vi "Save File Max Size Runtime.vi"(8 "Error In":errorcluster, 10 "File Size":dbl=5.0 format="%#_13g", 11 "Old path":path=path "C:/Data/T0000567/15HL2345/T0000567_15HL2345_GSH3456__140V_WTNote_RTHot Rinse_LSMax2_Date_07_30_2015_Time_16_09.csv") -> (0 "Error Out":errorcluster, 2 "New File":bool, 3 "New Path":path=path "C:/Data/T0000567/15HL2345/T0000567_15HL2345_GSH3456__140V_WTNote_RTHot Rinse_LSMax2_Date_07_30_2015_Time_16_09_File23.csv")   [LabVIEW 2019, in "Save File.lvlib"]
uses:
  Save File.lvlib
panel:
  # "C:\\Data\\T0000567\\15HL2345\\T0000567_15HL2345_GSH3456__140V_WTNote_RTHot Rinse_LSMax2_Date_07_30_2015_Time_16_09.csv"
  # "Y:\\5C\\2016\\15HL2345\\201606\\20160629\\Inv and MC\\TR_T0001000_Lab_ID_15HL2345_Model_GSH_AmbT_50_RH_50_Date_06_29_2016_Time_15_41HEWHFile4_Inv and MC.csv"
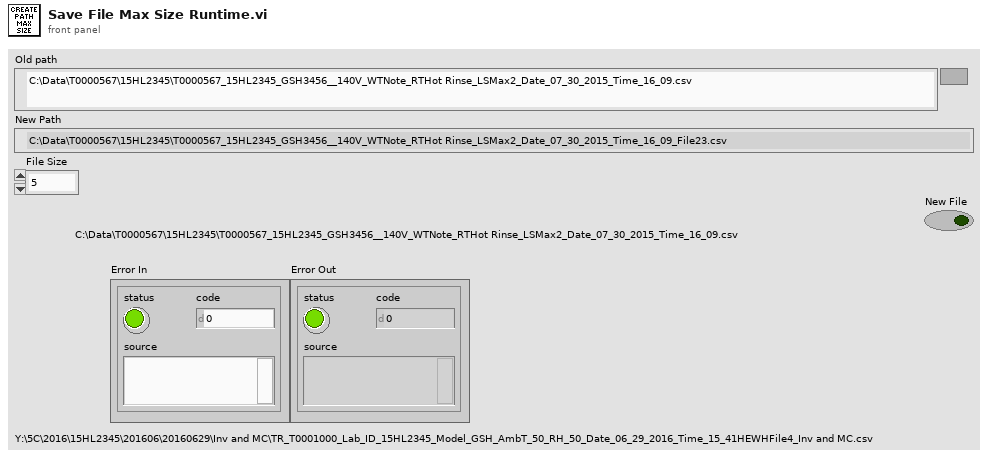
[diagram p1: front panel]
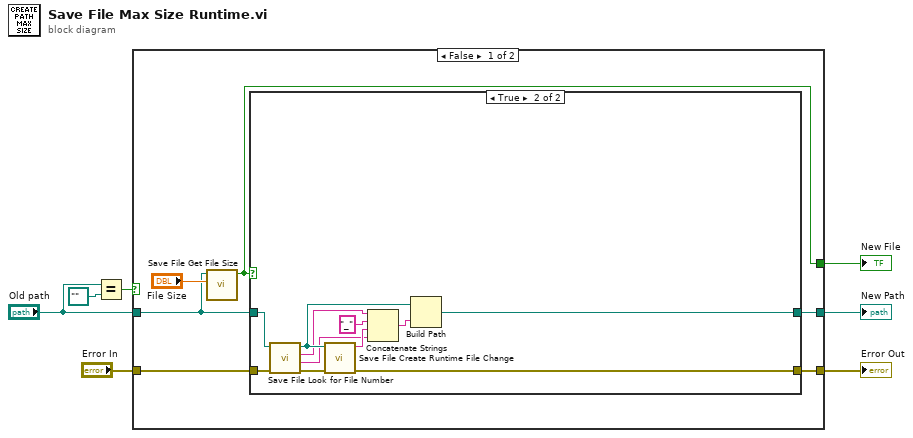
[diagram p0: block diagram]
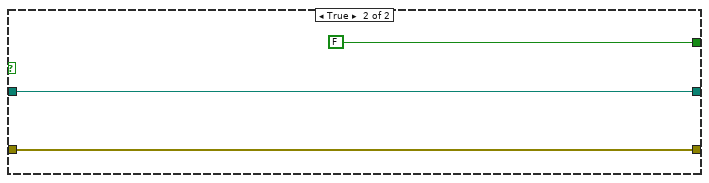
[diagram p3: hidden frame]
diagram:
  n1 = Equal?(x="Old path", y=path "") -> (x = y?=w4:bool)
  n2 = case shown="False" w4 {
    tunnel: [w12 w29] -> w7
    tunnel: "Old path" -> [w11 w29]
    tunnel: [w10 FALSE ("File Size Greater Than 5MB")] -> w3
    tunnel: "Error In" -> [w9 w27]
    tunnel: [w8 w27] -> w1
    frame False {
      n3 = call "Save File Get File Size.vi"("File Size"="File Size", "Old path"=w11) -> ("File Size Greater Than Limit"=w10:bool)  [unwired: 7 in, 2 out]
      n4 = case shown="True" w10 {
        tunnel: w11 -> [w15 w26]
        tunnel: [w15 w21] -> w12
        tunnel: w9 -> [w14 w18]
        tunnel: [w14 w16] -> w8
        frame False {
        }
        frame True {
          n5 = call "Save File Look for File Number.vi"("Error In"=w18, "Old path"=w26) -> ("Error Out"=w17:errorcluster, "Last Portion of File Name"=w19:string, "File Name (Before \"FILE\")"=w20:string, "Base Path (No File Name)"=w22:path)  [unwired: 6 in]
          n6 = call "Save File Create Runtime File Change.vi"("Error In"=w17, "Root Folder Path"=w22) -> ("Error Out"=w16:errorcluster, "File Number String"=w24:string)  [unwired: 8 in]
          n7 = Concatenate Strings(w20, "_" ("string"), w24, w19) -> (w23:string)
          n8 = Build Path(base path=w22, name or relative path=w23) -> (appended path=w21:path)
        }
      }
    }
    frame True {
    }
  }
  "New Path" <- w7
  "New File" <- w3
  "Error Out" <- w1
